vi "process controller save method.vi"(6 "default or user":T6, 8 "error in (not an error)":errorcluster, 10 "Action":T9) -> (0 "error out":errorcluster, 1 "sensor &var names":string[](array[string]), 2 "State names":string[](array[string]), 5 "output descriptions out":string[][](array[string]))   [LabVIEW 2019]
uses:
  file/file action.ctl
  Plant method.ctl
  operator info.ctl
  default or user select.ctl
  DAQ configuration/scale type.ctl
  calibration/correspondence table.ctl
  calibration/pH/pH scale.ctl
  calibration/Dissolved Oxygen/DO scale.ctl
  logic buffer cmd.ctl
  DAQ configuration/Sensor buffer command.ctl
  Calibration and Function folders.ctl
  calibration/Shared Data/share data command.ctl
panel:
  in  "Scale (prior to 11/12/15)":T5={"conversion matrix"=[[0.0, 0.0], [0.0, 0.0], [0.0, 0.0], [0.0, 0.0], [0.0, 0.0], [0.0, 0.0]], "units"="", "name"="", "scale type"=enum."Volts", "offset (volts)"=0.0, "second channel"=0, "correspondence table"=[], "offset (physical units)"=0.0, "pH scale"={"Buffers"=[], "Temperature"=0.0}, "D.O."={"Temperature"=0.0, "K"=0.0, "barometric pressure"=0.0}} {"D.O."."K" format="%.6f"; "D.O."."Temperature" format="%.2f"; "pH scale"."Buffers"."V/T" format="%.5f"; "pH scale"."Buffers"."Buffer" format="%.2f"; "pH scale"."Temperature" format="%.2f"; "offset (physical units)" format="%.5f"; "correspondence table"."volts" format="%.4f"; "correspondence table"."physical units" format="%.4f"; "second channel" min=-1; "offset (volts)" format="%.5f"; "conversion matrix" format="%.4e"}
  in  "Plant method in":T7={"Operator information"=[], "data log interval"=60, "data loop interval"=10, "Datalog directory path"=path "", "graph update interval"=1.0, "history length"=1000, "Control Logic file path"=path "", "Sensor Configuration file path"=path "", "HMI VI path"=path "", "HMI data smooth"=5.0} {"HMI data smooth" min=0.01 format="%.2f"; "history length" min=1; "graph update interval" min=0.001 format="%.2f"; "data log interval" min=1}
  # "C"
  # "kPa"
  # "C"
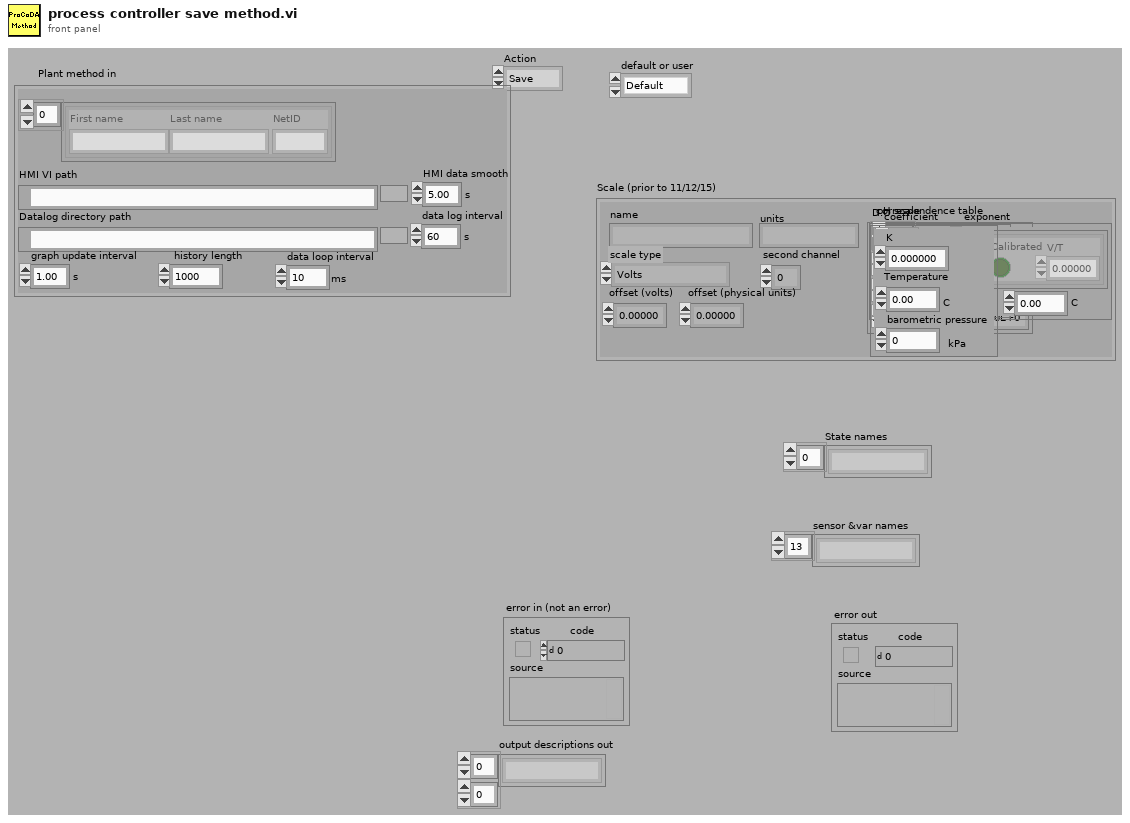
[diagram p1: front panel]
types:
  T1 = typedef "scale type.ctl" = enum16{"Volts", "Polynomial", "Correspondence Table", "pH", "Dissolved Oxygen", "Quadratic", "Photometer"}
  T2 = typedef "correspondence table.ctl" = cluster{"physical units":dbl, "volts":dbl}[]
  T3 = typedef "pH scale.ctl" = cluster{"Buffers":cluster{"Buffer":dbl, "Calibrated":bool, "V/T":dbl}[], "Temperature":dbl}
  T4 = typedef "DO scale.ctl" = cluster{"Temperature":dbl, "K":dbl, "barometric pressure":dbl}
  T5 = cluster{"conversion matrix":sgl[][], "units":string, "name":string, "scale type":T1, "offset (volts)":dbl, "second channel":i8, "correspondence table":T2, "offset (physical units)":dbl, "pH scale":T3, "D.O.":T4}
  T6 = typedef "default or user select.ctl" = enum16{"Default", "User select"}
  T7 = typedef "Plant method.ctl" = cluster{"Operator information":T8, "data log interval":u32, "data loop interval":u32, "Datalog directory path":path, "graph update interval":sgl, "history length":u16, "Control Logic file path":path, "Sensor Configuration file path":path, "HMI VI path":path, "HMI data smooth":dbl}
  T8 = typedef "operator info.ctl" = cluster{"First name":string, "Last name":string, "NetID":string}[]
  T9 = typedef "file action.ctl" = enum16{"Save", "Open"}
  T10 = typedef "share data command.ctl" = enum16{"Initialize from ini", "Update ini", "Write data", "Read data", "List my data", "List shared data", "Close"}
  T11 = typedef "Calibration and Function folders.ctl" = enum16{"Sensors", "Functions", "Config File", "PublicAppFolder", "New ini File", "Set Config File", "Delete ini File"}
  T12 = typedef "Sensor buffer command.ctl" = enum16{"read average", "read recent", "read all", "write", "set buffer size", "Read channel config", "Write channel config", "clear"}
  T13 = typedef "logic buffer cmd.ctl" = enum16{"read", "write ouput settings", "write rules", "write setpoints", "write output descriptions", "write all", "calculate setpoints", "save", "open", "Load all setpoint code", "Load one setpoint code", "Configure one setpoint code"}
  T14 = typedef "Channel config.ctl" = cluster{"Channel Indices":T15[], "AI Max voltage":dbl[], "Calibration matrix":T16}
  T15 = typedef "channel identifier.ctl" = u16
  T16 = typedef "calib array.ctl" = T17[]
  T17 = typedef "conversion.ctl" = cluster{"conversion matrix":sgl[][], "units":string, "name":string, "scale type":T1, "offset (volts)":dbl, "second channel":i8, "correspondence table":T2, "offset (physical units)":dbl, "pH scale":T3, "D.O.":T4, "Photometer data":T18}
  T18 = typedef "Photometer calibration data.ctl" = cluster{"Dark Voltage":dbl, "Blank Voltage":dbl, "Standards":cluster{"Concentration":dbl, "Voltage":dbl}[]}
  T19 = typedef "variable setpoint.ctl" = cluster{"name":string, "unit":string, "value":dbl, "Type":enum16{"Constant", "Variable"}, "variable":cluster{"selected sensors":i32[], "selected set points":i32[], "VI":path, "Data average interval":T20, "code ref":T21}}
  T20 = typedef "data ave interval.ctl" = dbl
  T21 = typedef "type specifier for control code.ctl" = refnum<vi>
  T22 = typedef "Output control.ctl" = u16[][]
  T23 = typedef "rules.ctl" = T24[]
  T24 = typedef "State rules.ctl" = cluster{"state rules":T25[], "State name":string}
  T25 = typedef "rule.ctl" = cluster{"next state":u16, "conditions":T26[], "number of conditions":u8, "Rule name":string}
  T26 = typedef "condition.ctl" = cluster{"> or <":T27, "set point":i32, "sensors and variables":i32, "Data average interval":dbl}
  T27 = typedef "greater or less.ctl" = bool
  T28 = cluster{"Calibration matrix":T16, "Channel Indices":T15[], "Set Points out":T19[], "ouput settings out":T22, "Rules out":T23, "output descriptions out":string[][]}
  T29 = cluster{"conversion matrix":sgl[][], "units":string, "name":string, "scale type":T1, "offset (volts)":dbl, "second channel":i8, "correspondence table":T2, "offset (physical units)":dbl, "pH scale":T3, "D.O.":T4}[]
  T30 = cluster{"Plant method in":T7, cluster{"conversion matrix":sgl[][], "units":string, "name":string, "scale type":T1, "offset (volts)":dbl, "second channel":i8, "correspondence table":T2, "offset (physical units)":dbl, "pH scale":T3, "D.O.":T4}[], "Channel Indices":T15[], "Set Points out":T19[], "ouput settings out":T22, "Rules out":T23, "output descriptions out":string[][]}
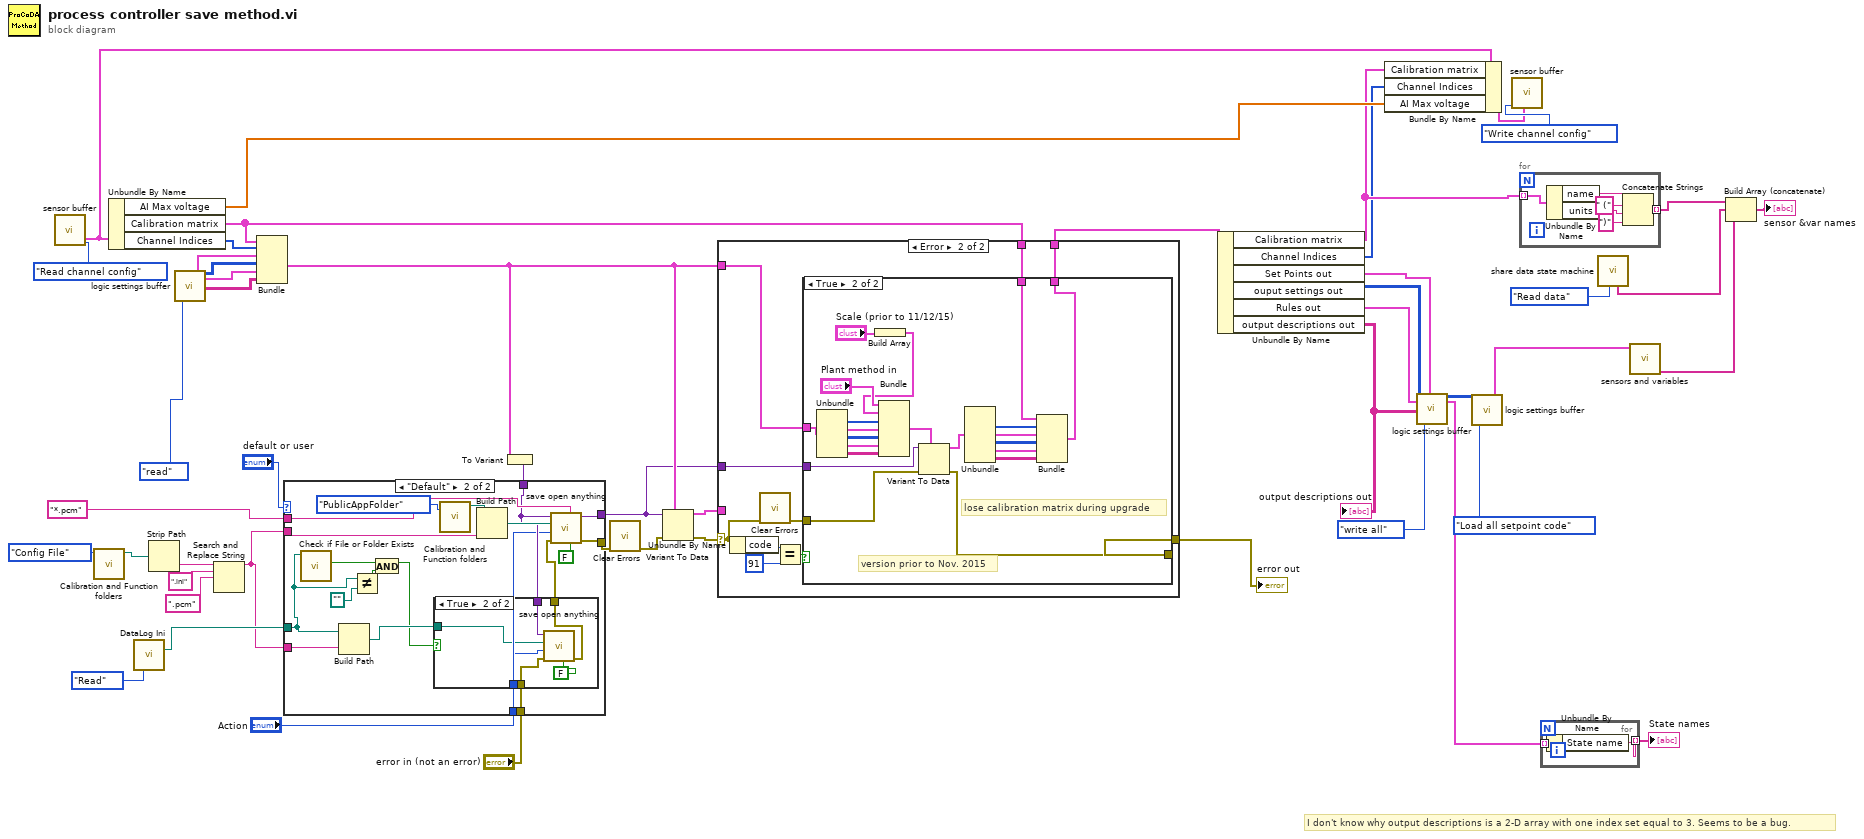
[diagram p0: block diagram]
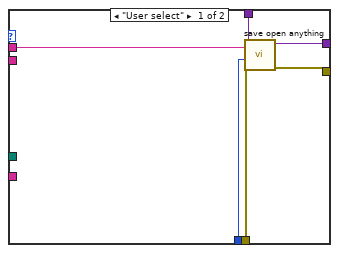
[diagram p2: hidden frame]
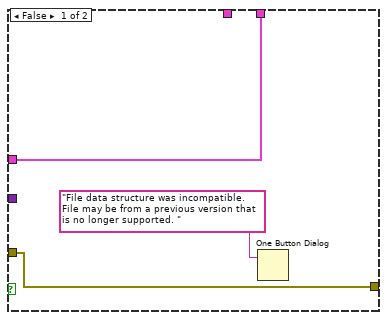
[diagram p5: hidden frame]
diagram:
  # "I don't know why output descriptions is a 2-D array with one index set equal to 3. Seems to be a bug."
  n1 = call "sensor buffer.vi"("command"=Sensor_buffer_command."Read channel config") -> ("Channel Config out"=w18:T14)  [unwired: 6 in, 4 out]
  n2 = call "Calibration and Function folders.vi"("Folder"=Calibration_and_Function_folders."Config File") -> ("Selected Folder"=w5:path)  [unwired: 9 in, 1 out]
  n3 = Unbundle By Name(w18) -> ("AI Max voltage"=w17:dbl[], "Calibration matrix"=w10:T16, "Channel Indices"=w20:T15[])
  n4 = call "DataLog Ini.vi"("Ini Cmd"=enum16{"Read", "Write"}."Read") -> ("Datalog directory path out"=w12:path)  [unwired: 9 in, 5 out]
  n5 = Strip Path(path=w5) -> (name=w9:string)  [unwired: 1 out]
  n6 = call "logic settings buffer.vi"("command"=logic_buffer_cmd."read") -> ("Set Points out"=w29:T19[], "ouput settings out"=w45:T22, "Rules out"=w44:T23, "output descriptions out"=w37:string[][])  [unwired: 11 in, 4 out]
  n7 = Search and Replace String(input string=w9, search string=".ini", replace string=".pcm" ("replace string (\"\")")) -> (result string=w6:string)  [unwired: 5 in, 3 out]
  n8 = Bundle("Calibration matrix"=w10, "Channel Indices"=w20, "Set Points out"=w29, "ouput settings out"=w45, "Rules out"=w44, "output descriptions out"=w37) -> (w25:T28)  [unwired: 1 in]
  n9 = To Variant(anything=w25) -> (Variant=w49:variant)
  n10 = case shown="\"Default\"" "default or user" {
    tunnel: "Action" -> [w56 w68]
    tunnel: w49 -> [w55 w69]
    tunnel: "error in (not an error)" -> [w54 w70]
    tunnel: [w53 w74] -> w47
    tunnel: "*.pcm" ("pattern") -> [w51 w72]
    tunnel: [w52 w75] -> w24
    tunnel: w12 -> [_ w63]
    tunnel: w6 -> [_ w60]
    tunnel: w6 -> [_ w59]
    frame "User select" {
      n11 = call "save open anything.vi"("Variant"=w55, "Action"=w56, "error in (not an error)"=w54, "pattern"=w51) -> ("Variant out"=w52:variant, "error out"=w53:errorcluster)  [unwired: 3 in, 2 out]
    }
    frame "Default" {
      n12 = call <vilib>:"Check if File or Folder Exists.vi"("path"=w63) -> ("file or folder exists?"=w67:bool)  [unwired: 8 in, 2 out]
      n13 = Build Path(base path=w63, name or relative path=w59) -> (appended path=w65:path)
      n14 = Not Equal?(x=w63, y=path "") -> (x != y?=w61:bool)
      n15 = And(x=w67, y=w61) -> (x .and. y?=w62:bool)
      n16 = case shown="True" w62 {
        tunnel: w70 -> [w76 w82]
        tunnel: w69 -> [_ w81]
        tunnel: w68 -> [_ w80]
        tunnel: w65 -> [_ w79]
        tunnel: [w76 w77] -> w66
        frame False {
        }
        frame True {
          n17 = call "save open anything.vi"("Variant"=w81, "file path"=w79, "Action"=w80, "error in (not an error)"=w82, "advisory dialog? (display:T)"=FALSE) -> ("error out"=w77:errorcluster)  [unwired: 2 in, 3 out]
        }
      }
      n18 = call "Calibration and Function folders.vi"("Folder"=Calibration_and_Function_folders."PublicAppFolder") -> ("Selected Folder"=w57:path)  [unwired: 9 in, 1 out]
      n19 = Build Path(base path=w57, name or relative path=w60) -> (appended path=w73:path)
      n20 = call "save open anything.vi"("Variant"=w69, "file path"=w73, "Action"=w68, "error in (not an error)"=w66, "pattern"=w72, "advisory dialog? (display:T)"=FALSE) -> ("Variant out"=w75:variant, "error out"=w74:errorcluster)  [unwired: 1 in, 2 out]
    }
  }
  n21 = call <vilib>:"Clear Errors.vi"("error in (no error)"=w47) -> ("error out"=w46:errorcluster)  [unwired: 5 in, 1 out]
  n22 = Variant To Data(error in=w46, type=w25, Variant=w24) -> (data=w31:T28, error out=w33:errorcluster)
  n23 = case shown="Error" w33 {
    selector: w33 -> [w83 w88]
    tunnel: [w84 w89] -> w32
    tunnel: w25 -> [_ w91]
    tunnel: w31 -> [w84 _]
    tunnel: w24 -> [_ w90]
    tunnel: [w83 w86] -> w11
    tunnel: w10 -> [_ w85]
    frame No Error {
    }
    frame Error {
      n24 = Unbundle By Name(w88) -> ("code"=w94:i32)
      n25 = call <vilib>:"Clear Errors.vi"("error in (no error)"=w88) -> ("error out"=w87:errorcluster)  [unwired: 5 in, 1 out]
      n26 = Equal?(x=w94, y=91) -> (x = y?=w92:bool)
      n27 = case shown="True" w92 {
        tunnel: w91 -> [w96 w118]
        tunnel: w90 -> [_ w116]
        tunnel: [w96 w110] -> w89
        tunnel: w87 -> [w95 w103]
        tunnel: [w95 w102] -> w86
        tunnel: w85 -> [_ w98]
        frame False {
          n28 = One Button Dialog(message="File data structure was incompatible. File may be from a previous version that is no longer supported. ") -> ()  [unwired: 1 in, 1 out]
        }
        frame True {
          # "lose calibration matrix during upgrade"
          # "version prior to Nov. 2015"
          n29 = Unbundle(w118) -> ("Channel Indices"=w109:T15[], "Set Points out"=w108:T19[], "ouput settings out"=w107:T22, "Rules out"=w106:T23, "output descriptions out"=w105:string[][])  [unwired: 1 out]
          n30 = Build Array("Scale (prior to 11/12/15)") -> (w99:T29)
          n31 = Bundle("Plant method in"="Plant method in", w99, "Channel Indices"=w109, "Set Points out"=w108, "ouput settings out"=w107, "Rules out"=w106, "output descriptions out"=w105) -> (w117:T30)  [unwired: 1 in]
          n32 = Variant To Data(error in=w103, type=w117, Variant=w116) -> (data=w113:T30, error out=w102:errorcluster)
          n33 = Unbundle(w113) -> ("Channel Indices"=w104:T15[], "Set Points out"=w114:T19[], "ouput settings out"=w115:T22, "Rules out"=w111:T23, "output descriptions out"=w112:string[][])  [unwired: 2 out]
          n34 = Bundle("Calibration matrix"=w98, "Channel Indices"=w104, "Set Points out"=w114, "ouput settings out"=w115, "Rules out"=w111, "output descriptions out"=w112) -> (w110:T28)  [unwired: 1 in]
        }
      }
    }
  }
  "error out" <- w11
  n35 = Unbundle By Name(w32) -> ("Calibration matrix"=w16:T16, "Channel Indices"=w15:T15[], "Set Points out"=w23:T19[], "ouput settings out"=w43:T22, "Rules out"=w42:T23, "output descriptions out"=w36:string[][])
  "output descriptions out" <- w36
  n36 = Bundle By Name(cluster=w18, "Calibration matrix"=w16, "Channel Indices"=w15, "AI Max voltage"=w17) -> (w14:T14)
  n37 = call "logic settings buffer.vi"("output settings"=w43, "Rules"=w42, "output descriptions"=w36, "command"=logic_buffer_cmd."write all", "Set Points"=w23) -> ("ouput settings out"=w35:T22, "Rules out"=w41:T23)  [unwired: 7 in, 6 out]
  n38 = call "logic settings buffer.vi"("output settings"=w35, "command"=logic_buffer_cmd."Load all setpoint code") -> ("Set Points out"=w26:T19[])  [unwired: 10 in, 7 out]
  n39 = call "sensor buffer.vi"("Channel Config"=w14, "command"=Sensor_buffer_command."Write channel config") -> ()  [unwired: 5 in, 5 out]
  n40 = for {
    tunnel: w16 -> [w124] mode=indexing
    tunnel: [w119] -> w28 mode=indexing
    n41 = Unbundle By Name(w124) -> ("name"=w123:string, "units"=w121:string)
    n42 = Concatenate Strings(w123, " (" ("string"), w121, ")" ("string")) -> (w119:string)
  }
  n43 = for {
    tunnel: w41 -> [w126] mode=indexing
    tunnel: [w125] -> w40 mode=indexing
    n44 = Unbundle By Name(w126) -> ("State name"=w125:string)
  }
  "State names" <- w40
  n45 = call "share data state machine.vi"("Share data command"=share_data_command."Read data") -> ("Shared data names (unit)"=w1:string[])  [unwired: 4 in, 6 out]
  n46 = call "sensors and variables.vi"("S P & V definitions"=w26) -> ("name (unit)"=w2:string[])  [unwired: 6 in, 4 out]
  n47 = Build Array (concatenate)(w28, w1, w2) -> (→"sensor &var names":string[])
